vi "format property to string line.vi"(2 "error in":errorcluster, 3 "Value":dbl format="%#_13g", 4 "Property":string="property", 5 "initial string":string) -> (0 "error out":errorcluster, 1 "resulting string":string)   [LabVIEW 2017, in "Magnet module.lvlib"]
uses:
  Magnet module.lvlib
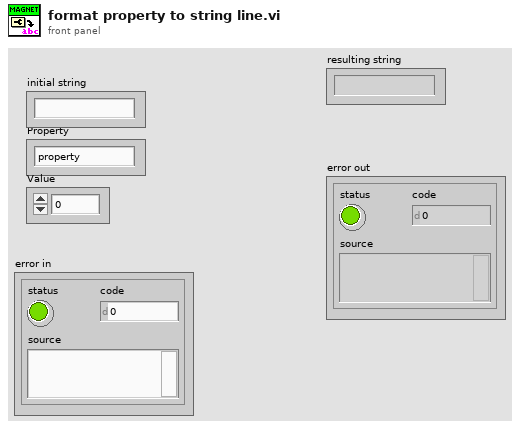
[diagram p1: front panel]
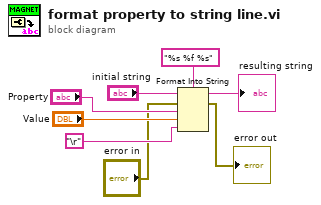
[diagram p0: block diagram]
diagram:
  n1 = Format Into String(format string="%s %f %s", initial string="initial string", error in="error in", "Property", "Value", "\r") -> (resulting string=→"resulting string":string, error out=→"error out":errorcluster)
